vi "edittest write sequence to file.vi"(6 "Spartan Version":T1 {"Build Date/Time" format="%<%X\n%x>T"}, 8 "error in (no error)":errorcluster, 10 "Sequence Record":T3, 11 "File Refnum In":T2) -> (0 "error out":errorcluster, 3 "File Refnum Out":T2)   [LabVIEW 2011]
uses:
  <vilib>/Utility/config.llb/Config Data RefNum.ctl
  server/database/Sequences/Sequence Record.ctl
  SI.LIB/OGAB Version.ctl
  <vilib>/Utility/config.llb/Write Key (String).vi
  <vilib>/Utility/config.llb/Write Key (I32).vi
  <vilib>/Utility/config.llb/Write Key (Boolean).vi
  <vilib>/Utility/config.llb/Write Key (Double).vi
  <vilib>/Utility/config.llb/NI_LVConfig.lvlib
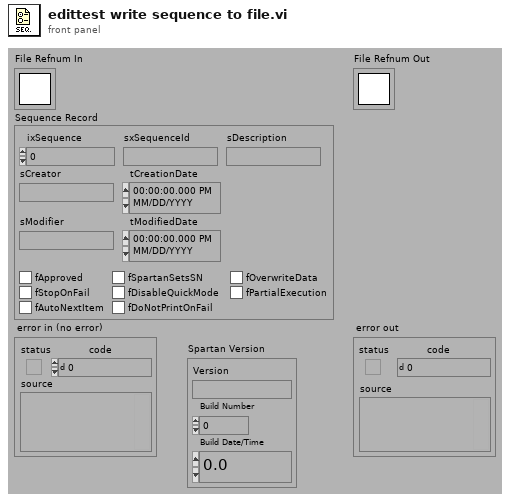
[diagram p1: front panel]
types:
  T1 = typedef "OGAB Version.ctl" = cluster{"Version":string, "Build Number":u32, "Build Date/Time":dbl}
  T2 = typedef "NI_LVConfig.lvlib/Config Data RefNum.ctl" = refnum<k1>
  T3 = typedef "Sequence Record.ctl" = cluster{"ixSequence":i32, "sxSequenceId":string, "sDescription":string, "sCreator":string, "tCreationDate":timestamp, "sModifier":string, "tModifiedDate":timestamp, "fApproved":bool, "fSpartanSetsSN":bool, "fOverwriteData":bool, "fStopOnFail":bool, "fDisableQuickMode":bool, "fPartialExecution":bool, "fAutoNextItem":bool, "fDoNotPrintOnFail":bool}
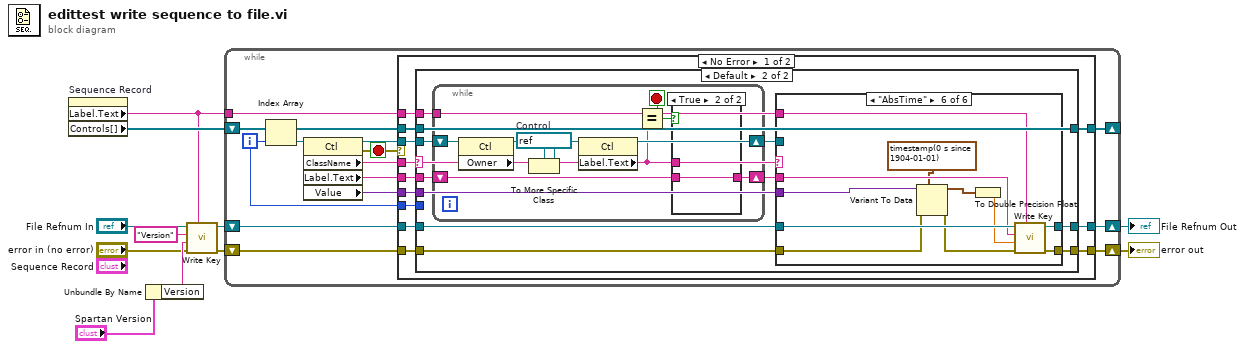
[diagram p0: block diagram]
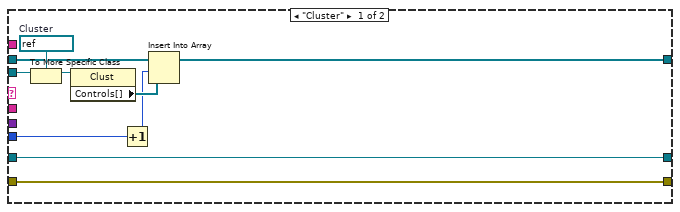
[diagram p2: hidden frame]
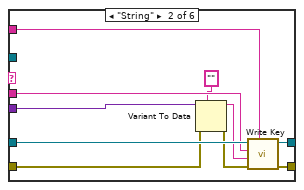
[diagram p4: hidden frame]
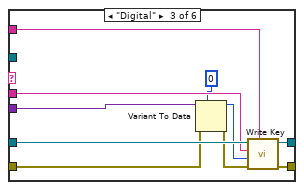
[diagram p5: hidden frame]
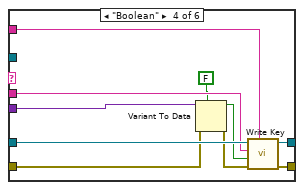
[diagram p6: hidden frame]
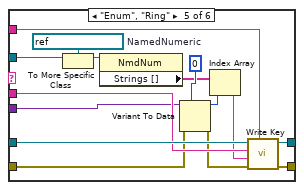
[diagram p7: hidden frame]
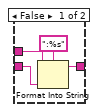
[diagram p8: hidden frame]
diagram:
  n1 = property on="Sequence Record" class="Clust (strict)"() -> ("Label.Text"=w6:string, "Controls[]"=w11:refnum<vi>[])  [unwired: 2 in, 2 out]
  n2 = Unbundle By Name("Spartan Version") -> ("Version"=w5:string)
  n3 = call-poly <vilib>:"Write Key.vi"("section"=w6, "error in (no error)"="error in (no error)", "value"=w5, "key"="Version", "refnum"="File Refnum In") -> ("error out"=w8:errorcluster, "refnum out"=w7:T2)  [unwired: 1 in, 4 out]
  n4 = while {
    shift-right: [w19] -> _
    shift-left: w11 -> [w21]
    shift-right: [w16] -> w10
    shift-left: w8 -> [w17]
    shift-right: [w15] -> w9
    shift-left: w7 -> [w18]
    tunnel: w6 -> [w14]
    i -> [w20]
    stop <- w23 stop-if-true
    n5 = Index Array(array=w21, index=w20) -> (element=w24:refnum<vi>)
    n6 = property class="Ctl"(reference=w24) -> (reference out=w22:refnum<vi>, error out=w23:errorcluster, "ClassName"=w13:string, "Label.Text"=w25:string, "Value"=w12:variant)  [unwired: 1 in]
    n7 = case shown="No Error" w23 {
      tunnel: w25 -> [w31 _]
      tunnel: w22 -> [w37 _]
      tunnel: w21 -> [w36 w134]
      tunnel: w20 -> [w35 _]
      tunnel: [w34 w134] -> w19
      tunnel: w18 -> [w30 w133]
      tunnel: w17 -> [w29 w132]
      tunnel: [w27 w132] -> w16
      tunnel: [w28 w133] -> w15
      tunnel: w14 -> [w33 _]
      tunnel: w13 -> [w32 _]
      tunnel: w12 -> [w26 _]
      frame No Error {
        n8 = case shown="Default" w32 {
          selector: w32 -> [_ w56]
          tunnel: w37 -> [w47 w48]
          tunnel: w36 -> [w44 w58]
          tunnel: w35 -> [w42 _]
          tunnel: [w40 w58] -> w34
          tunnel: w33 -> [_ w50]
          tunnel: w31 -> [_ w57]
          tunnel: w30 -> [w39 w55]
          tunnel: w29 -> [w38 w54]
          tunnel: [w39 w53] -> w28
          tunnel: [w38 w52] -> w27
          tunnel: w26 -> [_ w49]
          frame "Cluster" {
            w45 = refnum<vi> refnum  # Cluster
            n9 = To More Specific Class(target class=w45, reference=w47) -> (specific class reference=w46:refnum<vi>)  [unwired: 1 in, 1 out]
            n10 = property class="Clust"(reference=w46) -> ("Controls[]"=w43:refnum<vi>[])  [unwired: 1 in, 2 out]
            n11 = Increment(x=w42) -> (x+1=w41:i32)
            n12 = Insert Into Array(array=w44, index=w41, new element=w43) -> (w40:refnum<vi>[])
          }
          frame Default {
            n13 = while {
              shift-right: [w125] -> _
              shift-left: w48 -> [w126]
              tunnel: w50 -> [w121]
              shift-right: [w118] -> w51
              shift-left: w57 -> [w119]
              stop <- w120 stop-if-true
              w124 = refnum<vi> refnum  # Control
              n14 = property class="Ctl"(reference=w126) -> ("Owner"=w123:refnum<vi>)  [unwired: 1 in, 2 out]
              n15 = To More Specific Class(target class=w124, reference=w123) -> (specific class reference=w122:refnum<vi>)  [unwired: 1 in, 1 out]
              n16 = property class="Ctl"(reference=w122) -> (reference out=w125:refnum<vi>, "Label.Text"=w117:string)  [unwired: 1 in, 1 out]
              n17 = Equal?(x=w121, y=w117) -> (x = y?=w120:bool)
              n18 = case shown="True" w120 {
                tunnel: w119 -> [w127 w131]
                tunnel: [w129 w131] -> w118
                tunnel: w117 -> [w128 _]
                frame False {
                  n19 = Format Into String(format string=":%s", initial string=w128, w127) -> (resulting string=w129:string)  [unwired: 1 in, 1 out]
                }
                frame True {
                }
              }
            }
            n20 = case shown="\"AbsTime\"" w56 {
              tunnel: w55 -> [w60 w70 w80 w90 w105 w116]
              tunnel: w54 -> [w59 w63 w73 w83 w98 w110]
              tunnel: [w60 w69 w79 w89 w104 w115] -> w53
              tunnel: [w59 w68 w78 w88 w103 w114] -> w52
              tunnel: w51 -> [_ w67 w77 w87 w102 w113]
              tunnel: w50 -> [_ w66 w76 w86 w101 w112]
              tunnel: w49 -> [_ w65 w75 w85 w100 w111]
              tunnel: w48 -> [_ _ _ _ w95 _]
              frame Default {
              }
              frame "String" {
                n21 = Variant To Data(error in=w63, type="" ("format string"), Variant=w65) -> (data=w61:string, error out=w62:errorcluster)
                n22 = call-poly <vilib>:"Write Key.vi"("section"=w66, "error in (no error)"=w62, "value"=w61, "key"=w67, "refnum"=w70) -> ("error out"=w68:errorcluster, "refnum out"=w69:T2)  [unwired: 1 in, 4 out]
              }
              frame "Digital" {
                n23 = Variant To Data(error in=w73, type=0 ("format string"), Variant=w75) -> (data=w71:i32, error out=w72:errorcluster)
                n24 = call-poly <vilib>:"Write Key.vi"("section"=w76, "error in (no error)"=w72, "value"=w71, "key"=w77, "refnum"=w80) -> ("error out"=w78:errorcluster, "refnum out"=w79:T2)  [unwired: 5 out]
              }
              frame "Boolean" {
                n25 = Variant To Data(error in=w83, type=FALSE, Variant=w85) -> (data=w81:bool, error out=w82:errorcluster)
                n26 = call-poly <vilib>:"Write Key.vi"("section"=w86, "error in (no error)"=w82, "value"=w81, "key"=w87, "refnum"=w90) -> ("error out"=w88:errorcluster, "refnum out"=w89:T2)  [unwired: 5 out]
              }
              frame "Enum", "Ring" {
                w96 = refnum<vi> refnum  # NamedNumeric
                n27 = To More Specific Class(target class=w96, reference=w95) -> (specific class reference=w94:refnum<vi>)  [unwired: 1 in, 1 out]
                n28 = property class="NmdNum"(reference=w94) -> ("Strings []"=w93:string[])  [unwired: 1 in, 2 out]
                n29 = Variant To Data(error in=w98, type=0, Variant=w100) -> (data=w92:i32, error out=w97:errorcluster)
                n30 = Index Array(array=w93, index=w92) -> (element=w91:string)
                n31 = call-poly <vilib>:"Write Key.vi"("section"=w101, "error in (no error)"=w97, "value"=w91, "key"=w102, "refnum"=w105) -> ("error out"=w103:errorcluster, "refnum out"=w104:T2)  [unwired: 1 in, 4 out]
              }
              frame "AbsTime" {
                n32 = Variant To Data(error in=w110, type=timestamp(0 s since 1904-01-01), Variant=w111) -> (data=w107:timestamp, error out=w109:errorcluster)
                n33 = To Double Precision Float(number=w107) -> (double precision float=w106:dbl)
                n34 = call-poly <vilib>:"Write Key.vi"("section"=w112, "error in (no error)"=w109, "value"=w106, "key"=w113, "refnum"=w116) -> ("error out"=w114:errorcluster, "refnum out"=w115:T2)  [unwired: 3 in, 2 out]
              }
            }
          }
        }
      }
      frame Error {
      }
    }
  }
  "error out" <- w10
  "File Refnum Out" <- w9
